vi "ReplaceColor.vi"(5 "Replace color":fxp<+,3,3>, 7 "Color to replace":fxp<+,3,3>, 11 "color in":fxp<+,3,3>) -> (3 "color out":fxp<+,3,3>)   [LabVIEW 2019, in "GameEngine.lvlib"]
uses:
  GameEngine.lvlib
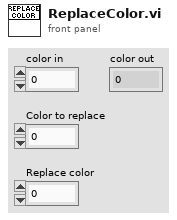
[diagram p1: front panel]
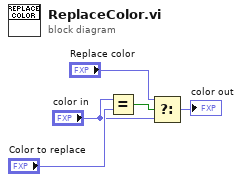
[diagram p0: block diagram]
diagram:
  n1 = Equal?(x="color in", y="Color to replace") -> (x = y?=w1:bool)
  n2 = Select(t="Replace color", s=w1, f="color in") -> (s? t:f=→"color out":fxp<+,3,3>)
